vi "ManualControl.vi"() -> ()   [LabVIEW 2012]
panel:
  in  "stop":bool
  in  "X axis 1":sgl(slide) scale=-1.0..1.0
  in  "Y axis 1":sgl(slide) scale=-1.0..1.0
  in  "X axis 2":sgl(slide) scale=-1.0..1.0
  in  "Y axis 2":sgl(slide) scale=-1.0..1.0
  in  "Triggers":sgl(slide) scale=-1.0..1.0
  out "pov 1":i32
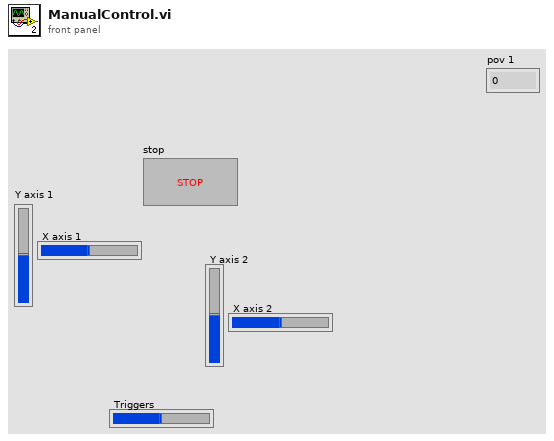
[diagram p1: front panel]
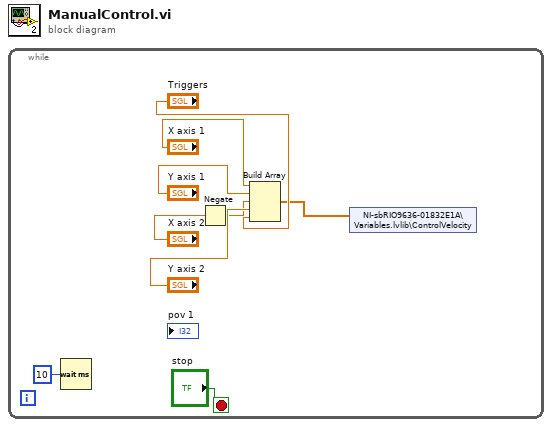
[diagram p0: block diagram]
diagram:
  n1 = while {
    stop <- "stop" stop-if-true
    n2 = Wait (ms)(milliseconds to wait=u32 10) -> ()  [unwired: 1 out]
    n3 = Negate(x="X axis 2") -> (-x=w1:sgl)
    n4 = Build Array("X axis 1", "Y axis 1", w1, "Y axis 2", "Triggers") -> (w3:sgl[])
    n5 = shared-variable "NI-sbRIO9636-01832E1A\\Variables.lvlib\\ControlVelocity"(w3) -> ()  [unwired: 1 in, 1 out]
  }
